vi "20211001_00.vi"() -> ()   [LabVIEW 2019]
panel:
  out "運轉中":bool
  in  "Ready":bool
  in  "停止":bool
  in  "啟動":bool
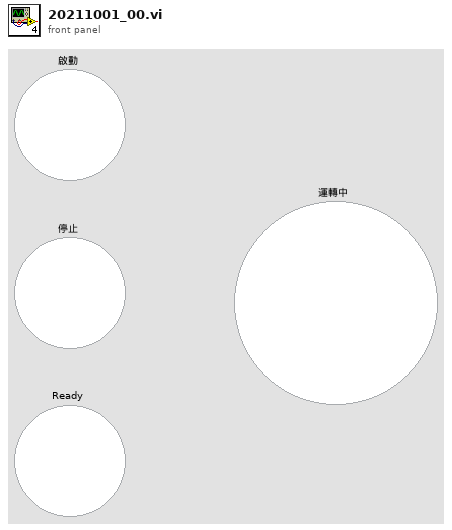
[diagram p1: front panel]
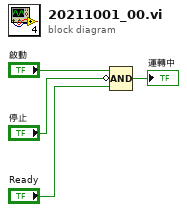
[diagram p0: block diagram]
diagram:
  n1 = Compound Arithmetic op=AND("啟動", invert "停止", "Ready") -> (→"運轉中":bool)
